vi "21 Talking Serial.vi"() -> ()   [LabVIEW 2024]
uses:
  <userlib>/1. Examples/_Subs/OpenDiagram/Open_XControl.xctl
  <vilib>/Instr/_visa.llb/VISA Configure Serial Port (Instr).vi
panel:
  in  "Stop Button":bool
  out "Console":string
  in  "Data to write":string
  in  "VISA resource name":refnum<visa-resource-name>
  in  "OpenDiag":refnum<vi>(xcontrol)
  # "01 Talking Serial\nThis code is a very simple terminal emulator\n\nInstructions:\n1. Select the desired serial port\n2. Hit Run and try it out (note that it will send your text and a '\\n')"
  # "Hit return when done typing"
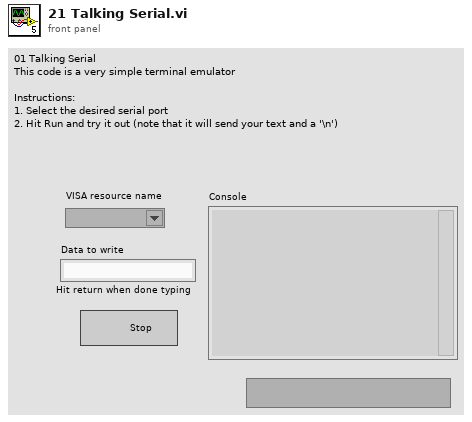
[diagram p1: front panel]
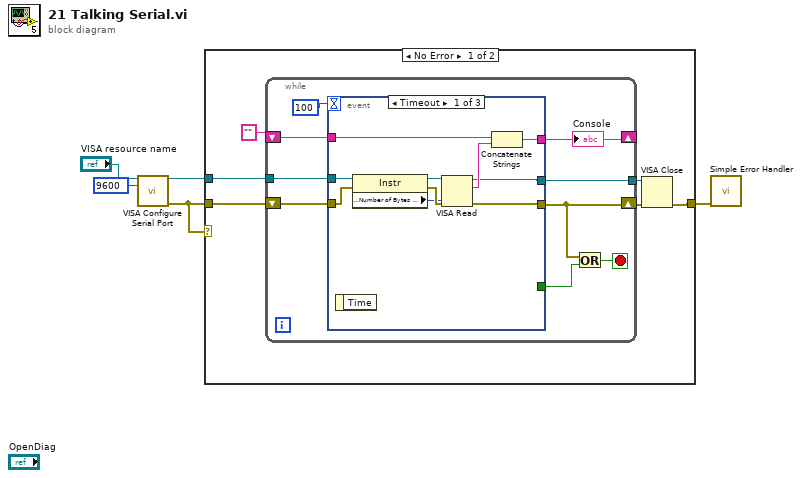
[diagram p0: block diagram]
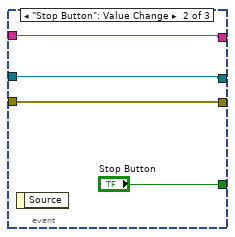
[diagram p2: hidden frame]
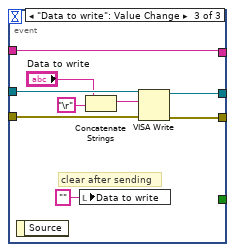
[diagram p3: hidden frame]
diagram:
  n1 = call-poly "VISA Configure Serial Port"("VISA resource name"="VISA resource name", "baud rate (9600)"=u32 9600) -> ("VISA resource name out"=w3:refnum<visa-resource-name>, "error out"=w2:errorcluster)  [unwired: 12 in]
  n2 = case shown="No Error" w2 {
    tunnel: w3 -> [w11 _]
    tunnel: w2 -> [w10 w44]
    tunnel: [w6 w44] -> w1
    frame No Error {
      n3 = while {
        tunnel: w11 -> [w20]
        shift-right: [w15] -> w7
        shift-left: w10 -> [w19]
        shift-right: [w16] -> _
        shift-left: "" -> [w17]
        tunnel: [w12] -> w8
        stop <- w13 stop-if-true
        n4 = event shown="[0] Timeout" {
          selector: _ -> [_ _ _]
          dyn-events: _ -> [_ _ _]
          timeout: 100 -> [_ _ _]
          tunnel: w20 -> [w30 w31 w43]
          tunnel: w19 -> [w29 w33 w42]
          tunnel: [w25 w33 w41] -> w15
          tunnel: w17 -> [w24 w32 w40]
          tunnel: [w22 w32 w40] -> w16
          tunnel: [_ "Stop Button" _] -> w14
          tunnel: [w21 w31 w38] -> w12
          event Timeout {
            n5 = event-data() -> ()  [unwired: 1 in, 1 out]
            n6 = property class="Instr"(reference=w30, error in=w29) -> (reference out=w26:refnum<visa-resource-name>, error out=w28:errorcluster, "Serial Settings:Number of Bytes at Serial Port"=w27:u32)
            n7 = VISA Read(VISA resource name=w26, byte count=w27, error in (no error)=w28) -> (VISA resource name out=w21:refnum<visa-resource-name>, read buffer=w23:string, error out=w25:errorcluster)  [unwired: 1 out]
            n8 = Concatenate Strings(w24, w23) -> (w22:string)
          }
          event "Stop Button": Value Change {
            n9 = event-data() -> ()  [unwired: 1 in, 1 out]
          }
          event "Data to write": Value Change {
            # "clear after sending"
            n10 = event-data() -> ()  [unwired: 1 in, 1 out]
            n11 = local write "Data to write"("" ("Data to write")) -> ()
            n12 = Concatenate Strings("Data to write", "\r") -> (w36:string)
            n13 = VISA Write(VISA resource name=w43, write buffer=w36, error in (no error)=w42) -> (VISA resource name out=w38:refnum<visa-resource-name>, error out=w41:errorcluster)  [unwired: 1 out]
          }
        }
        "Console" <- w16
        n14 = Or(x=w15, y=w14) -> (x .or. y?=w13:bool)
      }
      n15 = VISA Close(VISA resource name=w8, error in (no error)=w7) -> (error out=w6:errorcluster)
    }
    frame Error {
    }
  }
  n16 = call <vilib>:"Simple Error Handler.vi"("error in (no error)"=w1) -> ()  [unwired: 4 in, 5 out]
